vi "Pre Launch Init.vi"(11 "Automation Controller in":refnum<class "Automation Controller.lvclass">) -> (0 "error out":errorcluster, 3 "Automation Controller out":refnum<class "Automation Controller.lvclass">)   [LabVIEW 2024]
doc: "<p>(<strong>Filename</strong>: <span class=\"dnl\">Actor Framework.lvlib:Actor.lvclass:Pre Launch Init.vi</span>)</p>\n<p>Defines behavior that occurs after the <a href=\"nihelplauncher://docs/csh?context=lvcore_lvcomm_af_launch_nested_actor\">Launch Nested Actor</a> method is invoked but before the actor's Actor Core method begins running.</p>\n<p>By default, this method does nothing. A descendant class may override it to define behavior.</p>"
uses:
  Automation Controller.lvclass/Automation Controller.ctl
  Idle/Idle/Idle.lvclass
  Automation Controller.lvclass
  C:/Users/uspoaotto/OneDrive - Oregon Tool/Desktop/working copies/stateMachineActor/src/Automation Controller/Automation Controller/Automation Controller.lvclass
  C:/Users/uspoaotto/OneDrive - Oregon Tool/Desktop/working copies/stateMachineActor/src/State Machine Actor/State Machine Actor/State Machine Actor.lvclass
  C:/Users/uspoaotto/OneDrive - Oregon Tool/Desktop/working copies/stateMachineActor/src/_State Machine Actor/_State Machine Actor/_State Machine Actor.lvclass
  C:/Program Files (x86)/National Instruments/LabVIEW 2024/vi.lib/ActorFramework/Actor/Actor.lvclass
  C:/Users/uspoaotto/OneDrive - Oregon Tool/Desktop/working copies/stateMachineActor/src/Idle/Idle/Idle.lvclass
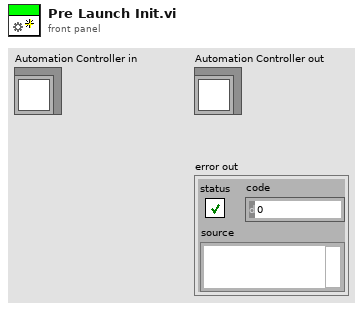
[diagram p1: front panel]
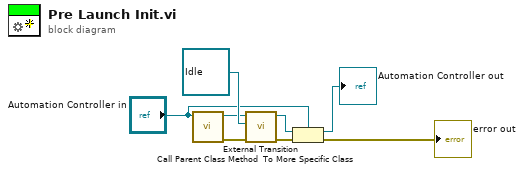
[diagram p0: block diagram]
diagram:
  n1 = call-parent "Call Parent Class Method"("_State Machine Actor in"="Automation Controller in") -> ("error out"=w3:errorcluster, "_State Machine Actor out"=w7:refnum<class "Automation Controller.lvclass">)  [unwired: 9 in]
  n2 = call-dynamic "External Transition.vi"("error in (no error)"=w3, "Target State"=refnum<class "Idle.lvclass"> refnum ("Idle.lvlib:Idle.lvclass"), "State Machine Actor in"=w7) -> ("error out"=w2:errorcluster, "_State Machine Actor out"=w5:refnum<class "_State Machine Actor.lvclass">)  [unwired: 7 in]
  n3 = To More Specific Class(target class="Automation Controller in", reference=w5, error in=w2) -> (specific class reference=→"Automation Controller out":refnum<class "Automation Controller.lvclass">, error out=→"error out":errorcluster)
